vi "FMPA Feed Bullseye.vi"(8 "Perfect circle XY bulls-eye":cluster{dbl[], dbl[]}(graph), 9 "Perfect circle?":bool, 10 "Init?":bool, 11 "POS array":dbl[](array[numeric])) -> (3 "Input XY bulls-eye":cluster{dbl[], dbl[]}(graph))   [LabVIEW 2023]
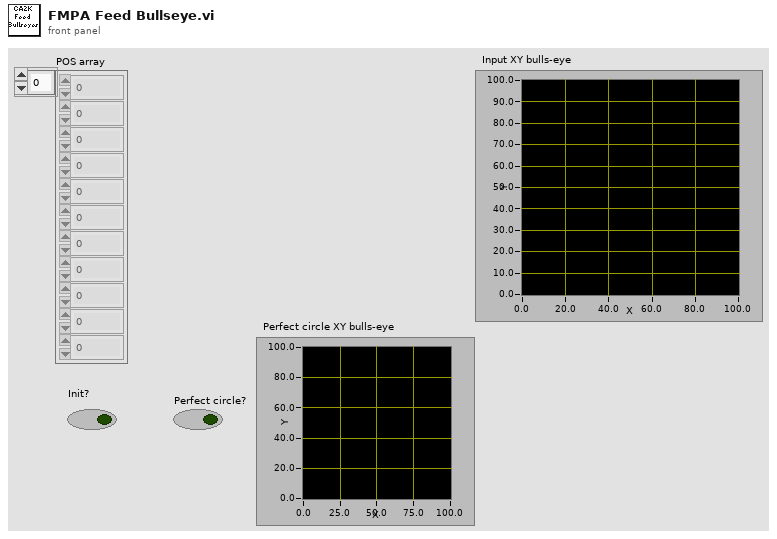
[diagram p1: front panel]
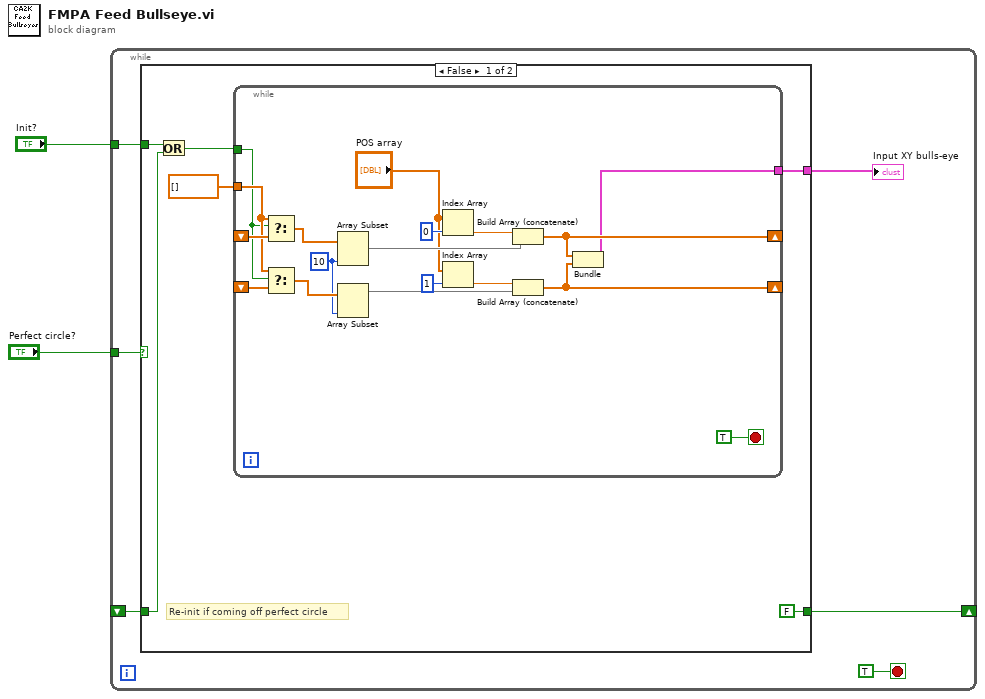
[diagram p0: block diagram]
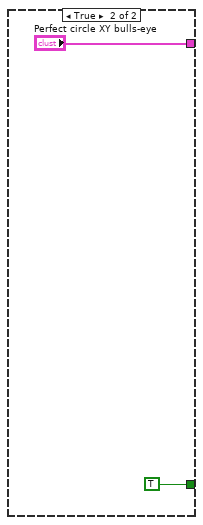
[diagram p2: hidden frame]
diagram:
  n1 = while {
    tunnel: "Perfect circle?" -> [w7]
    tunnel: "Init?" -> [w6]
    shift-right: [w5] -> _
    shift-left: _ -> [w3]
    stop <- TRUE stop-if-true
    n2 = case shown="False" w7 {
      tunnel: [w13 "Perfect circle XY bulls-eye"] -> w8
      tunnel: w6 -> [w11 _]
      tunnel: [FALSE TRUE] -> w5
      tunnel: w3 -> [w10 _]
      frame False {
        # "Re-init if coming off perfect circle"
        n3 = Or(x=w11, y=w10) -> (x .or. y?=w9:bool)
        n4 = while {
          shift-right: [w27] -> _
          shift-left: _ -> [w23]
          shift-right: [w26] -> _
          shift-left: _ -> [w21]
          tunnel: dbl[] [] -> [w20]
          tunnel: w9 -> [w19]
          tunnel: [w15] -> w13
          stop <- TRUE stop-if-true
          w17 = 10 ("length")
          n5 = Select(t=w20, s=w19, f=w23) -> (s? t:f=w22:dbl[])
          n6 = Select(t=w20, s=w19, f=w21) -> (s? t:f=w18:dbl[])
          n7 = Array Subset(array=w22, length=w17) -> (w29:dbl[])  [unwired: 1 in]
          n8 = Array Subset(array=w18, length=w17) -> (w16:dbl[])  [unwired: 1 in]
          n9 = Index Array(array="POS array", index=0) -> (element=w30:dbl)
          n10 = Index Array(array="POS array", index=1) -> (element=w28:dbl)
          n11 = Build Array (concatenate)(w30, w29) -> (w27:dbl[])
          n12 = Build Array (concatenate)(w28, w16) -> (w26:dbl[])
          n13 = Bundle(w27, w26) -> (w15:cluster{dbl[], dbl[]})  [unwired: 1 in]
        }
      }
      frame True {
      }
    }
    "Input XY bulls-eye" <- w8
  }
